vi "Write Routines.vi"(8 "error in (no error)":errorcluster, 10 "Routines":refnum<class "Routine.lvclass">[](array[class]), 11 "Assembly Run in":refnum<class "Assembly Run.lvclass">) -> (0 "error out":errorcluster, 3 "Assembly Run out":refnum<class "Assembly Run.lvclass">)   [LabVIEW 2016, in "Assembly Run.lvclass"]
uses:
  Assembly Run.lvclass
  Routine/Routine.lvclass
  Assembly Run.lvclass/Assembly Run.ctl
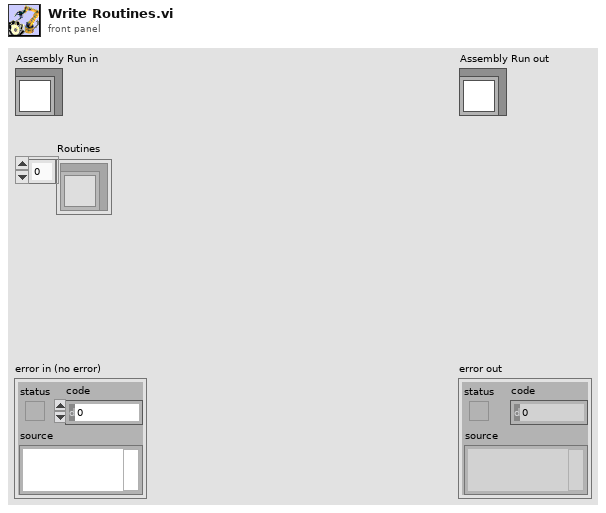
[diagram p1: front panel]
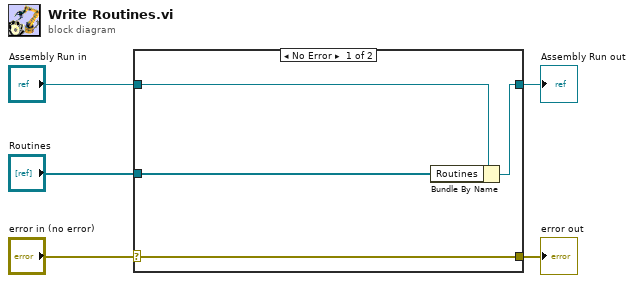
[diagram p0: block diagram]
diagram:
  n1 = case shown="No Error" "error in (no error)" {
    selector: "error in (no error)" -> [w9 w10]
    tunnel: [w9 w10] -> w4
    tunnel: [w7 w11] -> w2
    tunnel: "Assembly Run in" -> [w8 w11]
    tunnel: "Routines" -> [w6 _]
    frame No Error {
      n2 = Bundle By Name(cluster=w8, "Routines"=w6) -> (w7:refnum<class "Assembly Run.lvclass">)
    }
    frame Error {
    }
  }
  "error out" <- w4
  "Assembly Run out" <- w2
